vi "1_Channel_Trigger_and_FIFO.vi"(6 "data in":T1={"channel 0"=[0.0, 0.0], "channel 1"=[0.0, 0.0], "channel 2"=[0.0, 0.0], "channel 3"=[0.0, 0.0], "channel 4"=[0.0, 0.0], "channel 5"=[0.0, 0.0], "channel 6"=[0.0, 0.0], "channel 7"=[0.0, 0.0]}, 7 "Channel":i8, 9 "Trig Cfg":T3, 10 "FIFO Cfg":T7, 11 "Status":T2) -> (1 "Trigger Index":u16, 2 "TrigCount":u32, 3 "TrigCfg":T8, 4 "overflow":bool)   [LabVIEW 2021]
doc: "All Trigger and FIFO functions for one channel.\nLuke Graham 12-28-2022"
uses:
  Controls/Clust/WindowTriggerClust.ctl
  <instrlib>/_niInstr/Data Trigger/v1/Shared/Public/Level Configuration FXP(+-,18,1).ctl
  <instrlib>/_niInstr/Data Trigger/v1/Shared/Public/Level Configuration Trigger When.ctl
  Controls/Clust/All_acquisition_Resources.ctl
  <instrlib>/_niInstr/Multirecord Acquisition/Common/v1/FPGA/niInstr Multirecord Acquisition Common v1 FPGA.lvclass
  C:/Program Files (x86)/National Instruments/LabVIEW 2021/instr.lib/_niInstr/Multirecord Acquisition/Interface/v1/FPGA/niInstr Multirecord Acquisition v1 FPGA.lvclass
  Controls/Clust/Trig_Config_Clust.ctl
  Host/Clusts/AllWindowsClust.ctl
  Host/Clusts/ChannelWindowClust.ctl
  FPGA Interface Typedefinitions/Trigger Combination Type.ctl
  Controls/Clust/Status_Booleans_Clust.ctl
  Trigger/SubVIs/Types/Trigger Type.ctl
  <instrlib>/_niInstr/Data Trigger/v1/Shared/Public/Edge Configuration FXP(+-,18,1).ctl
  <instrlib>/_niInstr/Data Trigger/v1/Shared/Public/Edge Configuration Trigger Slope.ctl
  Controls/Clust/Update_Trigger_Center.ctl
  <instrlib>/_niInstr/Basic Elements/v1/FPGA/Private/Count Up U32.vi
  Data Type Conversion/SubVIs/Remove Overflow FXP(+-,18,1)x8ch.vi
  Data Type Conversion/SubVIs/Data Type Conversion FXP(+-,18,1) to I16x8ch.vi
  <instrlib>/_niInstr/Channel/v1/FPGA/Private/Select and Interleave/Select And Interleave I16xNspcx8ch.vi
  <instrlib>/_niInstr/Multirecord Acquisition/Interface/v1/FPGA/Private/Write I16 Wrapper.vi
  Trigger/Trigger FXP(+,-,18,1).vi
  <instrlib>/_niInstr/Data Trigger/v1/Shared/niInstr Data Trigger v1 Shared.lvlib
  <instrlib>/_niInstr/Basic Elements/v1/FPGA/niInstr Basic Elements v1 FPGA.lvlib
  <instrlib>/_niInstr/Channel/v1/FPGA/niInstr Channel v1 FPGA.lvlib
  <instrlib>/_niInstr/Multirecord Acquisition/Interface/v1/FPGA/niInstr Multirecord Acquisition v1 FPGA.lvclass
  C:/Program Files (x86)/National Instruments/LabVIEW 2021/instr.lib/_niInstr/Multirecord Acquisition/Common/v1/FPGA/niInstr Multirecord Acquisition Common v1 FPGA.lvclass
  FPGA Interface Typedefinitions/FPGA Interface Typedefinitions.lvlib
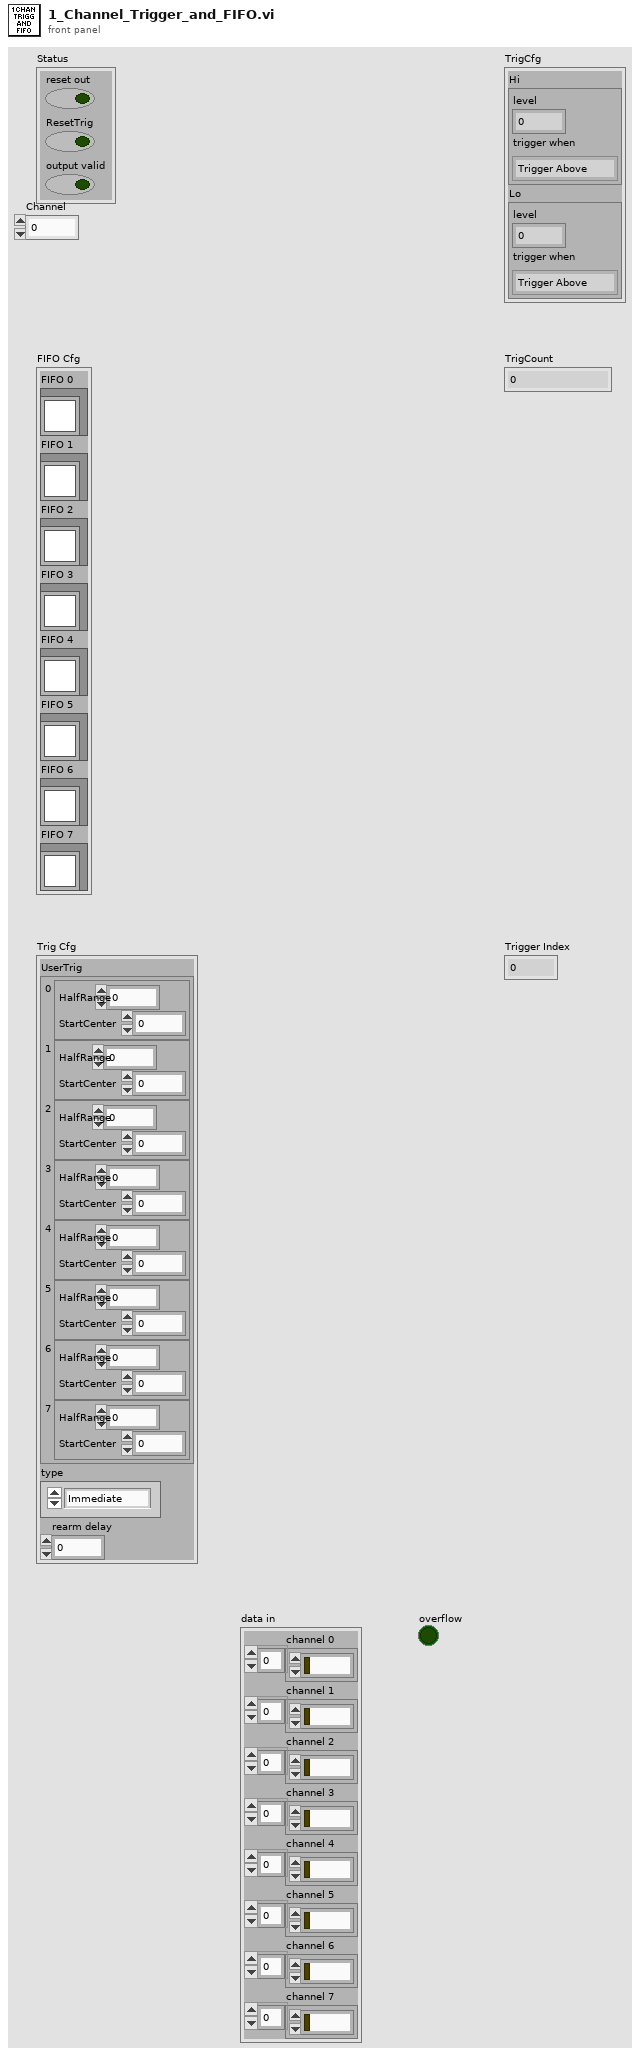
[diagram p1: front panel]
types:
  T1 = cluster{"channel 0":fxp<+/-,18,1>[], "channel 1":fxp<+/-,18,1>[], "channel 2":fxp<+/-,18,1>[], "channel 3":fxp<+/-,18,1>[], "channel 4":fxp<+/-,18,1>[], "channel 5":fxp<+/-,18,1>[], "channel 6":fxp<+/-,18,1>[], "channel 7":fxp<+/-,18,1>[]}
  T2 = typedef "Status_Booleans_Clust.ctl" = cluster{"reset out":bool, "ResetTrig":bool, "output valid":bool}
  T3 = typedef "Trig_Config_Clust.ctl" = cluster{"UserTrig":T4, "type":T6, "rearm delay":u16}
  T4 = typedef "AllWindowsClust.ctl" = cluster{"0":T5, "1":T5, "2":T5, "3":T5, "4":T5, "5":T5, "6":T5, "7":T5}
  T5 = typedef "ChannelWindowClust.ctl" = cluster{"HalfRange":fxp<+/-,18,5>, "StartCenter":fxp<+/-,18,5>}
  T6 = typedef "FPGA Interface Typedefinitions.lvlib/Trigger Combination Type.ctl" = enum16{"Immediate", "A", "B", "OR", "AND", "A THEN B", "B THEN A", "High Resolution"}
  T7 = typedef "All_acquisition_Resources.ctl" = cluster{"FIFO 0":refnum<class "niInstr Multirecord Acquisition Common v1 FPGA.lvclass">, "FIFO 1":refnum<class "niInstr Multirecord Acquisition Common v1 FPGA.lvclass">, "FIFO 2":refnum<class "niInstr Multirecord Acquisition Common v1 FPGA.lvclass">, "FIFO 3":refnum<class "niInstr Multirecord Acquisition Common v1 FPGA.lvclass">, "FIFO 4":refnum<class "niInstr Multirecord Acquisition Common v1 FPGA.lvclass">, "FIFO 5":refnum<class "niInstr Multirecord Acquisition Common v1 FPGA.lvclass">, "FIFO 6":refnum<class "niInstr Multirecord Acquisition Common v1 FPGA.lvclass">, "FIFO 7":refnum<class "niInstr Multirecord Acquisition Common v1 FPGA.lvclass">}
  T8 = typedef "WindowTriggerClust.ctl" = cluster{"Hi":T9, "Lo":T9}
  T9 = typedef "niInstr Data Trigger v1 Shared.lvlib/Level Configuration FXP(+-,18,1).ctl" = cluster{"level":fxp<+/-,18,5>, "trigger when":T10}
  T10 = typedef "niInstr Data Trigger v1 Shared.lvlib/Level Configuration Trigger When.ctl" = enum8{"Trigger Above", "Trigger Below"}
  T11 = typedef "Update_Trigger_Center.ctl" = cluster{"New Center":fxp<+/-,18,5>, "apply":bool}
  T12 = typedef "Trigger Type.ctl" = enum16{"Edge", "Level", "Custom"}
  T13 = typedef "niInstr Data Trigger v1 Shared.lvlib/Edge Configuration FXP(+-,18,1).ctl" = cluster{"highLevel":fxp<+/-,18,1>, "lowLevel":fxp<+/-,18,1>, "trigger slope":T14}
  T14 = typedef "niInstr Data Trigger v1 Shared.lvlib/Edge Configuration Trigger Slope.ctl" = enum8{"Positive", "Negative"}
  T15 = cluster{"channel 0":i16[], "channel 1":i16[], "channel 2":i16[], "channel 3":i16[], "channel 4":i16[], "channel 5":i16[], "channel 6":i16[], "channel 7":i16[]}
  T16 = typedef "niInstr Multirecord Acquisition v1 FPGA.lvclass/Timestamp.ctl" = cluster{"timestamp":u64, "valid":bool}
  T17 = typedef "niInstr Types v1 Shared.lvlib/Input Triggers.ctl" = cluster{"start":bool, "advance":bool, "reference":bool, "start trigger index":u16, "advance trigger index":u16, "reference trigger index":u16, "reference trigger correction cycle count":u32}
  T18 = typedef "All_Window_Triggers_Clust.ctl" = cluster{"0":T8, "1":T8, "2":T8, "3":T8, "4":T8, "5":T8, "6":T8, "7":T8}
  T19 = typedef "niInstr Types v1 Shared.lvlib/Sample Format.ctl" = cluster{"bits per channel":u16, "samples per clock":u16, "channels":u8}
  T20 = typedef "niInstr Multirecord Acquisition v1 FPGA.lvclass/Events.ctl" = cluster{"ready for start":bool, "ready for advance":bool, "ready for reference":bool, "end of record":bool, "done":bool, "start trigger":bool, "advance trigger":bool, "reference trigger":bool, "start trigger index":u16, "advance trigger index":u16, "reference trigger index":u16}
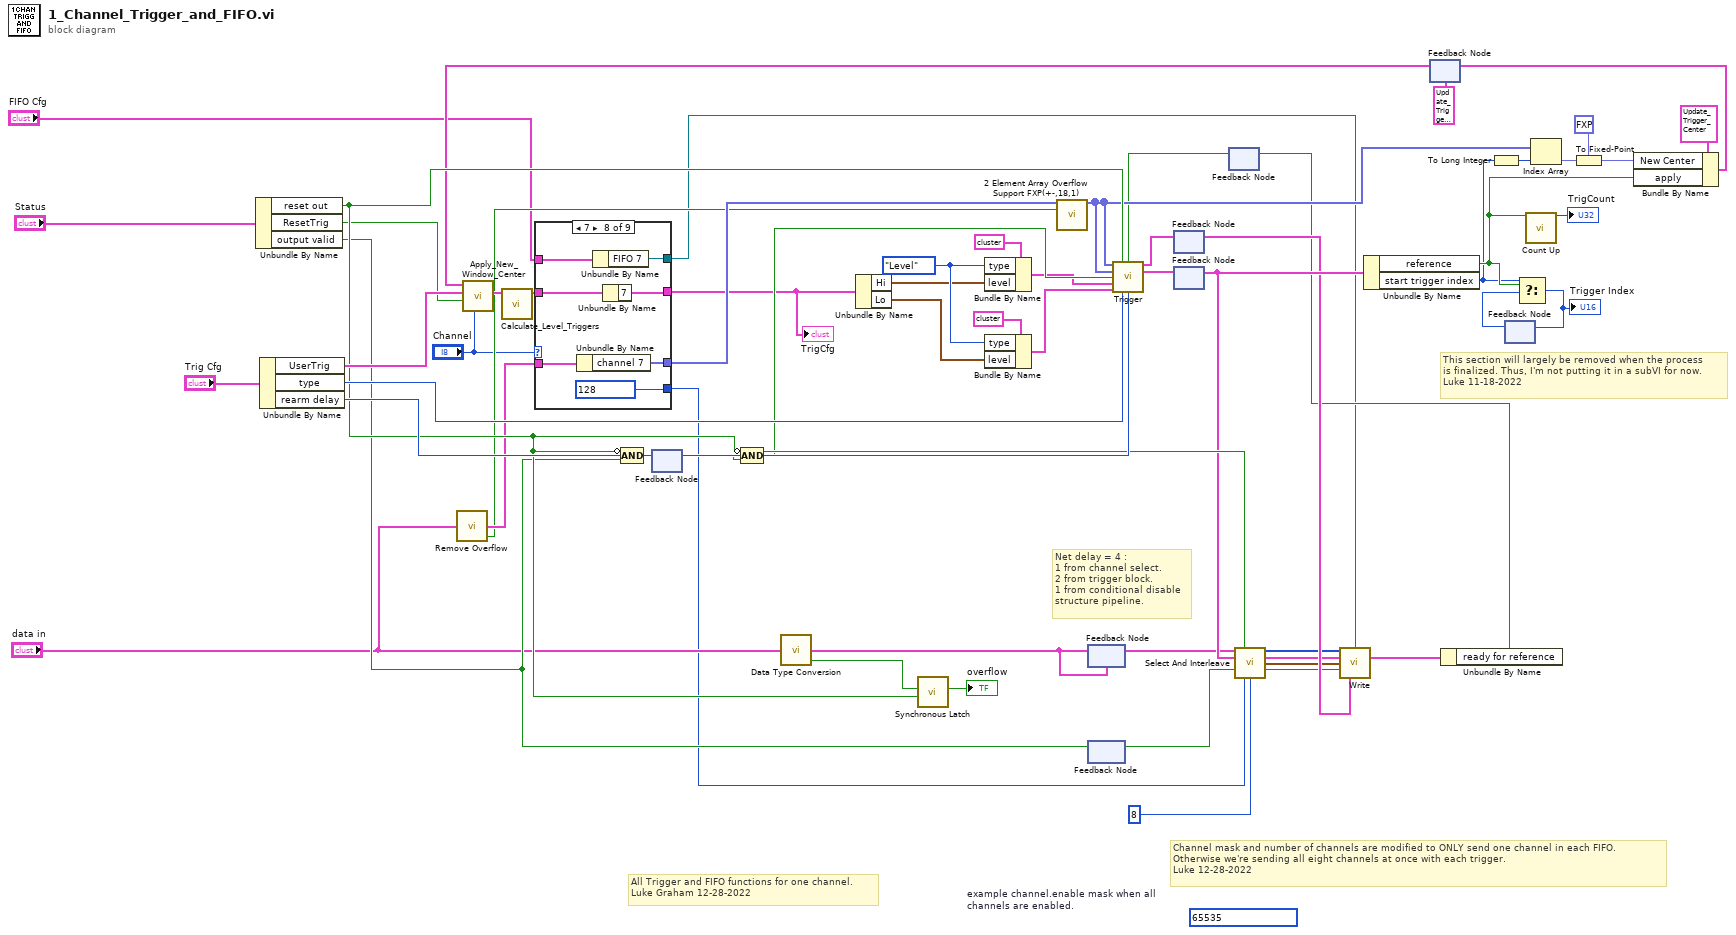
[diagram p0: block diagram]
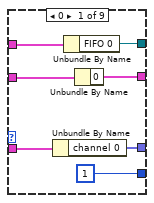
[diagram p2: hidden frame]
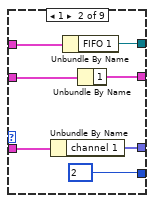
[diagram p3: hidden frame]
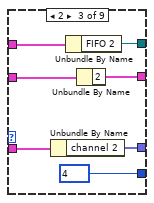
[diagram p4: hidden frame]
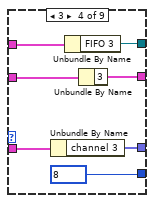
[diagram p5: hidden frame]
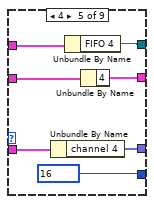
[diagram p6: hidden frame]
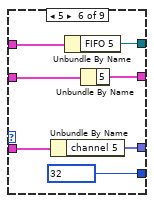
[diagram p7: hidden frame]
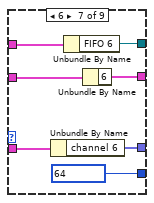
[diagram p8: hidden frame]
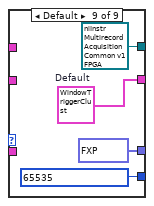
[diagram p9: hidden frame]
diagram:
  (unwired) u16 65535  # example channel.enable mask when all channels are enabled.
  w24 = Trigger_Type."Level" ("type")
  # "Channel mask and number of channels are modified to ONLY send one channel in each FIFO.\nOtherwise we're sending all eight channels at once with each trigger.\nLuke 12-28-2022"
  # "All Trigger and FIFO functions for one channel.\nLuke Graham 12-28-2022"
  # "This section will largely be removed when the process\nis finalized. Thus, I'm not putting it in a subVI for now.\nLuke 11-18-2022"
  # "Net delay = 4 :\n1 from channel select.\n2 from trigger block.\n1 from conditional disable structure pipeline."
  n1 = Unbundle By Name("Status") -> ("reset out"=w56:bool, "ResetTrig"=w54:bool, "output valid"=w55:bool)
  n2 = Unbundle By Name("Trig Cfg") -> ("UserTrig"=w58:T4, "type"=w59:T6, "rearm delay"=w60:u16)
  n3 = call-poly "Remove Overflow.vi"("data in"="data in") -> ("overflow"=w19:bool, "data out"=w30:T1)  [unwired: 3 in]
  n4 = Compound Arithmetic op=AND(invert w56, w55) -> (w28:bool)
  n5 = feedback #1() -> (w27:bool)  [unwired: 1 in]
  n6 = feedback-in #1(w28) -> ()
  n7 = Compound Arithmetic op=AND(invert w56, w27) -> (w29:bool)
  n8 = call-poly "Data Type Conversion.vi"("data in"="data in") -> ("overflow"=w32:bool, "data out"=w35:T15)  [unwired: 3 in]
  n9 = call <instrlib>:"Synchronous Latch.vi"("clear"=w56, "set"=w32) -> ("out"=→"overflow":bool)  [unwired: 9 in]
  n10 = feedback #2(w35) -> (w33:T15)
  n11 = feedback-in #2(w35) -> ()
  n12 = feedback #3() -> (w36:bool)  [unwired: 1 in]
  n13 = feedback-in #3(w55) -> ()
  n14 = feedback #4() -> (w26:T16)  [unwired: 1 in]
  n15 = feedback #5() -> (w37:T17)  [unwired: 1 in]
  n16 = feedback #6() -> (w14:bool)  [unwired: 1 in]
  n17 = Unbundle By Name(w37) -> ("reference"=w48:bool, "start trigger index"=w42:u16)
  n18 = feedback #7(T11 {"New Center"=0.0, "apply"=FALSE}) -> (w49:T11)
  n19 = call "Apply_New_Window_Center.vi"("Chan# (only Channel 0 works now)"="Channel", "ResetTrig"=w54, "User Trig"=w58, "FeedbackTrig"=w49) -> ("AllWindows out"=w52:T4)  [unwired: 7 in]
  n20 = call "Calculate_Level_Triggers.vi"("AllWindows"=w52) -> ("All_Window_Trigs"=w6:T18)  [unwired: 8 in, 2 out]
  n21 = case shown="7" "Channel" {
    tunnel: [w67 w74 w81 w88 w95 w102 w109 w116 fxp<+/-,18,1>[] [-1.0, 0.0] ("channel 7")] -> w31
    tunnel: w30 -> [w66 w73 w80 w87 w94 w101 w108 w115 _]
    tunnel: w6 -> [w65 w72 w79 w86 w93 w100 w107 w114 _]
    tunnel: [w64 w71 w78 w85 w92 w99 w106 w113 w118] -> w5
    tunnel: "FIFO Cfg" -> [w63 w70 w77 w84 w91 w98 w105 w112 _]
    tunnel: [w62 w69 w76 w83 w90 w97 w104 w111 refnum<class "niInstr Multirecord Acquisition Common v1 FPGA.lvclass"> refnum ("FIFO 7")] -> w3
    tunnel: [u16 1 ("channel.enable mask") u16 2 ("channel.enable mask") u16 4 ("channel.enable mask") u16 8 ("channel.enable mask") u16 16 ("channel.enable mask") u16 32 ("channel.enable mask") u16 64 ("channel.enable mask") u16 128 ("channel.enable mask") u16 65535 ("channel.enable mask")] -> w2
    frame 0 {
      n22 = Unbundle By Name(w66) -> ("channel 0"=w67:fxp<+/-,18,1>[])
      n23 = Unbundle By Name(w63) -> ("FIFO 0"=w62:refnum<class "niInstr Multirecord Acquisition Common v1 FPGA.lvclass">)
      n24 = Unbundle By Name(w65) -> ("0"=w64:T8)
    }
    frame 1 {
      n25 = Unbundle By Name(w73) -> ("channel 1"=w74:fxp<+/-,18,1>[])
      n26 = Unbundle By Name(w70) -> ("FIFO 1"=w69:refnum<class "niInstr Multirecord Acquisition Common v1 FPGA.lvclass">)
      n27 = Unbundle By Name(w72) -> ("1"=w71:T8)
    }
    frame 2 {
      n28 = Unbundle By Name(w80) -> ("channel 2"=w81:fxp<+/-,18,1>[])
      n29 = Unbundle By Name(w77) -> ("FIFO 2"=w76:refnum<class "niInstr Multirecord Acquisition Common v1 FPGA.lvclass">)
      n30 = Unbundle By Name(w79) -> ("2"=w78:T8)
    }
    frame 3 {
      n31 = Unbundle By Name(w87) -> ("channel 3"=w88:fxp<+/-,18,1>[])
      n32 = Unbundle By Name(w84) -> ("FIFO 3"=w83:refnum<class "niInstr Multirecord Acquisition Common v1 FPGA.lvclass">)
      n33 = Unbundle By Name(w86) -> ("3"=w85:T8)
    }
    frame 4 {
      n34 = Unbundle By Name(w94) -> ("channel 4"=w95:fxp<+/-,18,1>[])
      n35 = Unbundle By Name(w91) -> ("FIFO 4"=w90:refnum<class "niInstr Multirecord Acquisition Common v1 FPGA.lvclass">)
      n36 = Unbundle By Name(w93) -> ("4"=w92:T8)
    }
    frame 5 {
      n37 = Unbundle By Name(w101) -> ("channel 5"=w102:fxp<+/-,18,1>[])
      n38 = Unbundle By Name(w98) -> ("FIFO 5"=w97:refnum<class "niInstr Multirecord Acquisition Common v1 FPGA.lvclass">)
      n39 = Unbundle By Name(w100) -> ("5"=w99:T8)
    }
    frame 6 {
      n40 = Unbundle By Name(w108) -> ("channel 6"=w109:fxp<+/-,18,1>[])
      n41 = Unbundle By Name(w105) -> ("FIFO 6"=w104:refnum<class "niInstr Multirecord Acquisition Common v1 FPGA.lvclass">)
      n42 = Unbundle By Name(w107) -> ("6"=w106:T8)
    }
    frame 7 {
      n43 = Unbundle By Name(w115) -> ("channel 7"=w116:fxp<+/-,18,1>[])
      n44 = Unbundle By Name(w112) -> ("FIFO 7"=w111:refnum<class "niInstr Multirecord Acquisition Common v1 FPGA.lvclass">)
      n45 = Unbundle By Name(w114) -> ("7"=w113:T8)
    }
    frame Default {
      w118 = T8 {"Hi"={"level"=0.0, "trigger when"=enum."Trigger Above"}, "Lo"={"level"=0.0, "trigger when"=enum."Trigger Above"}}  # Default
    }
  }
  "TrigCfg" <- w5
  n46 = Unbundle By Name(w5) -> ("Hi"=w23:T9, "Lo"=w25:T9)
  n47 = Bundle By Name(cluster=cluster{"type":T12, "level":T9, "edge":T13} {"type"=enum."Edge", "level"={"level"=0.0, "trigger when"=enum."Trigger Above"}, "edge"={"highLevel"=0.0, "lowLevel"=0.0, "trigger slope"=enum."Positive"}} ("trigger.A"), "type"=w24, "level"=w23) -> (w17:cluster{"type":T12, "level":T9, "edge":T13})
  n48 = Bundle By Name(cluster=cluster{"type":T12, "level":T9, "edge":T13} {"type"=enum."Edge", "level"={"level"=0.0, "trigger when"=enum."Trigger Above"}, "edge"={"highLevel"=0.0, "lowLevel"=0.0, "trigger slope"=enum."Positive"}} ("trigger.A"), "type"=w24, "level"=w25) -> (w18:cluster{"type":T12, "level":T9, "edge":T13})
  n49 = call "2 Element Array Overflow Support FXP(+-,18,1).vi"("data in"=w31, "overflow"=w19) -> ("data out"=w41:fxp<+/-,18,1>[])  [unwired: 13 in]
  n50 = call-poly "Trigger.vi"("data A"=w41, "reset"=w56, "trigger.ready for reference"=w14, "data B"=w41, "input valid"=w29, "trigger.A"=w17, "trigger.B"=w18, "trigger.combination type"=w59, "rearm delay"=w60) -> ("timestamps"=w21:T16, "trigger.out"=w20:T17)  [unwired: 3 in, 2 out]
  n51 = feedback-in #4(w21) -> ()
  n52 = feedback-in #5(w20) -> ()
  n53 = call-poly <instrlib>:"Select And Interleave.vi"("data in"=w33, "reset"=w56, "triggers in"=w37, "input valid"=w36, "channel enable mask"=w2, "number of channels to interleave"=u8 8 ("channel.number of channels")) -> ("interleaved data out"=w8:i16[], "triggers out"=w9:T17, "sample format out"=w10:T19, "output valid"=w11:bool)  [unwired: 5 in, 1 out]
  n54 = call-poly <instrlib>:"Write.vi"("data"=w8, "acquisition resources"=w3, "triggers"=w9, "sample format"=w10, "data valid"=w11, "timestamp"=w26) -> ("events"=w12:T20)  [unwired: 6 in, 3 out]
  n55 = Unbundle By Name(w12) -> ("ready for reference"=w13:bool)
  n56 = feedback-in #6(w13) -> ()
  n57 = To Long Integer(number=w42) -> (32bit integer=w43:i32)
  n58 = feedback #8() -> (w40:u16)  [unwired: 1 in]
  n59 = Select(t=w42, s=w48, f=w40) -> (s? t:f=w39:u16)
  "Trigger Index" <- w39
  n60 = feedback-in #8(w39) -> ()
  n61 = call-poly <instrlib>:"Count Up.vi"("increment"=w48) -> ("count out"=→"TrigCount":u32)  [unwired: 14 in]
  n62 = Index Array(array=w41, index=w43) -> (element=w44:fxp<+/-,18,1>)
  n63 = To Fixed-Point(fixed-point type=fxp<+/-,18,5> 0.0, number=w44) -> (fixed-point=w47:fxp<+/-,18,5>)
  n64 = Bundle By Name(cluster=T11 {"New Center"=0.0, "apply"=FALSE}, "New Center"=w47, "apply"=w48) -> (w50:T11)
  n65 = feedback-in #7(w50) -> ()
